vi "ValueChangeTracker.vi"(11 "Data In":variant) -> (3 "Array":cluster{"Data In":variant, "Occurances":i32}[](array[cluster]))   [LabVIEW 2017]
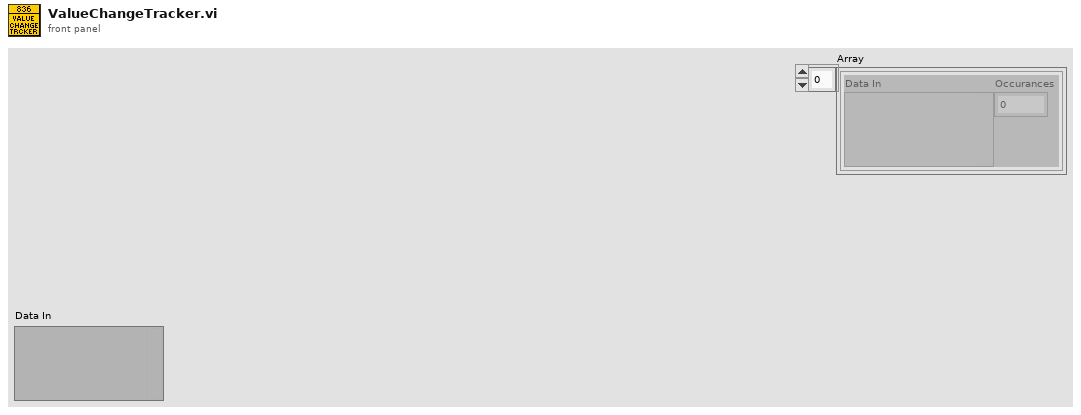
[diagram p1: front panel]
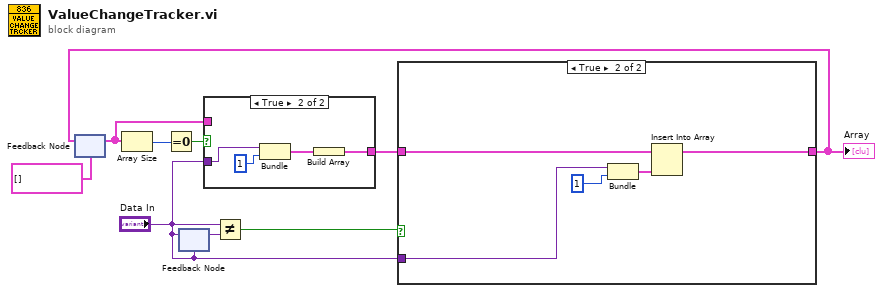
[diagram p0: block diagram]
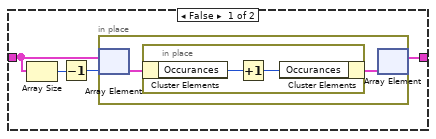
[diagram p2: hidden frame]
diagram:
  n1 = feedback #1(cluster{"Data":variant, "Occurances":i32}[] [] ("Array")) -> (w5:cluster{"Data":variant, "Occurances":i32}[])
  n2 = Array Size(array=w5) -> (size(s)=w7:i32)
  n3 = Equal To 0?(x=w7) -> (x = 0?=w6:bool)
  n4 = feedback-in #2("Data In") -> ()
  n5 = feedback #2("Data In") -> (w9:variant)
  n6 = case shown="True" w6 {
    tunnel: w5 -> [w10 _]
    tunnel: [w10 w12] -> w3
    tunnel: "Data In" -> [_ w14]
    frame False {
    }
    frame True {
      n7 = Bundle("Data In"=w14, 1) -> (w11:cluster{"Data In":variant, i32})  [unwired: 1 in]
      n8 = Build Array(w11) -> (w12:cluster{"Data In":variant, i32}[])
    }
  }
  n9 = Not Equal?(x="Data In", y=w9) -> (x != y?=w4:bool)
  n10 = case shown="True" w4 {
    tunnel: w3 -> [w18 w27]
    tunnel: "Data In" -> [_ w25]
    tunnel: [w15 w23] -> w1
    frame False {
      n11 = Array Size(array=w18) -> (size(s)=w17:i32)
      n12 = Decrement(x=w17) -> (x-1=w16:i32)
      n13 = in-place {
        n14 = in-place-array #3(w18, w16) -> (w20:cluster{"Data In":variant, "Occurances":i32})
        n15 = in-place {
          n16 = in-place-cluster #4(w20) -> ("Occurances"=w22:i32)
          n17 = Increment(x=w22) -> (x+1=w21:i32)
          n18 = in-place-cluster #4("Occurances"=w21) -> (w19:cluster{"Data In":variant, "Occurances":i32})
        }
        n19 = in-place-array #3(w19) -> (w15:cluster{"Data In":variant, "Occurances":i32}[])  [unwired: 1 out]
      }
    }
    frame True {
      n20 = Bundle("Data In"=w25, 1) -> (w24:cluster{"Data In":variant, i32})  [unwired: 1 in]
      n21 = Insert Into Array(array=w27, new element=w24) -> (w23:cluster{"Data In":variant, "Occurances":i32}[])  [unwired: 1 in]
    }
  }
  "Array" <- w1
  n22 = feedback-in #1(w1) -> ()
